vi "Process button press.vi"(0 "DataCluster in":T1={"JSONRead"={"ConfigurationFilePaths"={"Default JSON Path in"=path "", "Rack Controller Override JSON file path in"=path "", "Algorithm Overrride JSON file path in "=path ""}, "ConfigurationVariants"={"Default JSON \nVariant"=variant(cluster{"Inspection States":enum16{"PreSelect", "Back _Inspection", "Analytics", "Ready To Run", "Ready To Insert", "Enable All buttons", "Disable All Buttons", "Settings", "Select", "Stop", "Pause", "Inspect"}} {"Inspection States"=enum."PreSelect"}), "Algorithm Override\nJSON Variant"=variant(cluster{"Diagnostics States":enum16{"Enable All", "Camera Optics Fail", "Loading Bar", "Camera Optics", "Motor", "Arduino", "POST Done", "POST"}} {"Diagnostics States"=enum."Enable All"}), "Rack Controller Override\nJSON Variant"=variant(cluster{"Edit Limits":enum16{"Update List"}, "Enable Disable Measurements":enum16{"Back to Edit Tolerance"}, "Page Select":enum16{"Edit Tolerance Limits", "Enable Disable Buttons"}} {"Edit Limits"=enum."Update List", "Enable Disable Measurements"=enum."Back to Edit Tolerance", "Page Select"=enum."Edit Tolerance Limits"})}, "ConfigurationCluster"={"UIParameters"={"SpecificationVersion"="", "Title"="", "NumberOfImagesToBeDisplayed"=0.0, "ImageCountWindow"=0.0, "FontName"="", "FontSize"=0.0, "CustomerLogoFilePath"="", "ZentronLogoFilePath"="", "CompatibleSoftwareVersions"=[], "CameraLabelMapping"=[], "ImageIndicatorLayouts"=[], "SoftwareButtonLabels"={"SelectLabel"="", "RunLabel"="", "PauseLabel"="", "StopLabel"=""}, "DiagnosticsParameters"={"CameraOpticsDiagnostics"={"Label"="", "CameraLabelsList"=[]}, "ArduinoDiagnostics"={"Label"=""}, "MotorDiagnostics"={"Label"=""}, "ReelerMotor"={"Label"=""}, "TowerLampDiagnostics"={"Label"=""}, "TriggerSensor"={"Label"="", "SensorsList"=[]}, "HardwareButtonDiagnostics"={"Label"=""}, "MasterSampleDiagnostics"={"Label"=""}}, "DieIdParameters"={"DefaultDieId"="", "DieIdsList"=[]}, "EventReasonsList"={"Pause"=[], "Stop"=[], "FailPause"=[], "Ignored"=[], "DefaultEventReason"=""}, "StampingMachineIds"=[], "ErrorPopupStrings"=[]}}}, "Inspection"={"Inspection After Stop"=FALSE, "IsPaused"=FALSE, "Camera Names"=[], "Fail Array"=[], "Reel Number"=0, "Image details_init"=[], "LSL"=[], "USL"=[], "Max limits"={"Production max"=0, "Reel max"=0}, "parts List"=[], "#Racks"=0, "MeasurementNames"=[], "Reel complete"=FALSE, "Fail event reason list"=[]}, "Diagnostics"={"Selection Done?"=FALSE, "Diagnostics details"={"Diagnostics names"={"Main diagnostics"=[], "Sub diagnostics names"={"Camera optics"=[], "Trigger sensor"=[]}}, "Diagnostics labels"={"Main diagnostics"=[], "Sub diagnostics names"={"Camera optics"=[], "Trigger sensor"=[]}}}, "DiagnosticsFeatures"={"ArduinoDiagnostics"=FALSE, "MotorDiagnostics"=FALSE, "CameraOpticsDiagnostics"=FALSE, "ReelerMotor"=FALSE, "HardwareButtonDiagnostics"=FALSE, "TriggerSensor"=FALSE, "TowerLampDiagnostics"=FALSE, "MasterSampleDiagnostics"=FALSE}, "SelectedDiagnostics"=""}, "EditToleranceSettings"={"Input ListBox"={"Measurement Values"=[], "Cluster of Limits"={"LSL"=0.0, "USL"=0.0, "LCL"=0.0, "UCL"=0.0}, "Rack Selection"=enum."Both Racks", "M and N Array"=[], "Ticked Measurement Index"=[], "Measurements Enabled"=[], "Current Active Position"={"Horizontal"=0, "Vertical"=0}, "Current ticked measurement"=0.0}, "Saved?"=FALSE, "IsETLSelected"=FALSE, "IsPartSelected"=FALSE}, "ControlsIndicators"={"General"={"Main Tab"=refnum, "Inspection SubPanel_Inspection"=refnum, "Zen Logo_Inspection"=refnum, "SoftwareExit"=refnum, "Loading Bar VI Ref"=refnum, "Right Pane Tab"=refnum, "Image Reference array"=[], "Command tab"=refnum, "Inspection subTab control ref"=refnum, "SelectionCluster"={"ok"=refnum, "confirm"=refnum, "reset"=refnum, "change"=refnum, "TOTAL COUNT"=refnum, "REEL COUNT"=refnum, "PART NAME"=refnum, "VERIFIED"=refnum, "OPERATOR NAME"=refnum, "Select message"=refnum}, "Event  Reason  List"=refnum, "Event reason blink"=refnum, "Event reason switching tab"=refnum, "confirm_eventReason"=refnum}, "Inspection"={"Inspection Status"=refnum, "Run_Inspection"=refnum, "Pause_Inspection"=refnum, "Stop_Inspection"=refnum, "Settings_Inspection"=refnum, "Inspection Images VI Ref"=refnum, "Pass-Fail Indicator String"=refnum, "Analytics_Inspection"=refnum, "Label array"=[], "Analytics VI\nreference"=refnum, "Counts"=refnum, "Cards array"=refnum, "Counts array"=[]}, "Diagnostics"={"Diagnostics Tab"=refnum, "Dust indicator :"=refnum, "Logout_Diagnostics"=refnum, "CAMERA STATUS MESSAGE"=refnum, "BUZZER OFF"=refnum, "PAUSE"=refnum, "STOP"=refnum, "RUN"=refnum, "Current Diagnostics Status"=refnum, "Select a diagnostics"=refnum, "Diagnostics Status"=refnum, "Select a sub diagnostics"=refnum, "Optics img"=refnum, "Diagnostics Status\nString"=refnum}, "Edit Tolerance Limits"={"Tolerance Limits Listbox"=refnum, "Enable Disable"=refnum, "Cluster of limits"=refnum, "Thresholds limits"=refnum, "Update List"=refnum, "Save"=refnum, "Back_Edit Tolerance"=refnum, "logout"=refnum, "Select a part"=refnum, "Bias Correction"=refnum, "Linearity Correction"=refnum, "Select a Rack"=refnum, "ETS tab"=refnum, "Factory reset"=refnum, "Door\nPoka Yoke"=refnum, "Fail count reverse"=refnum, "ETL count error message"=refnum, "ETL help string"=refnum}, "Master sample"={"Master sample message"=refnum, "Master sample tab"=refnum, "Next"=refnum, "Repeat"=refnum, "Master sample part message"=refnum}}, "AdditionalFeatures"={"Cp Cpk details"={"CpCpkData"=[], "Cp Cpk popup"=refnum}, "Popup"={"Restore main tab"="", "Popup data"={"Loading bar data"={"Open?"=FALSE, "Display string"=""}, "Pop-up"={"Pop-up Type"=enum."Open Logo Display", "Title"="", "Message"="", "Button 1 Text"="", "Button 2 Text"="", "Show Close? T/F"=FALSE, "Title Blink? T/F"=FALSE, "Title Blink Colour"=0}}}, "DynamicImageHandling"={"Image update"=[], "RBCIA"=[], "ISIM"=[], "Camera labels list"=[], "Enable DIH?"=FALSE, "Init DIH params?"=FALSE}, "PageHandling"={"Previous State"={"Inspection"={"Inspection States"=enum."PreSelect"}, "Diagnostics"={"Diagnostics States"=enum."Enable All"}, "Edit Tolerance"={"Edit Limits"=enum."Update List", "Enable Disable Measurements"=enum."Back to Edit Tolerance", "Page Select"=enum."Edit Tolerance Limits"}, "Page Select"=enum."Edit Tolerance"}, "Current state"="", "Previous control access state"=""}, "Core"={"Current VI Reference"=refnum, "Close Panel on Exit?"=FALSE}, "SlaveLoopData"={"EnableShortKeyPress"=FALSE, "Point32"={"Horizontal"=0, "Vertical"=0}}, "Chosen event reason"="", "Master sample validation"={"Master sample general message"="", "Master sample part message"=""}, "Fail Ignore Count Reversal"={"Production ignored count"=0, "Reel ignored count"=0}}}, 1 "Label.Text":string, 5 "Send ClusterData":refnum<user-event>, 9 "Self Enqueuer":refnum<class "Message Enqueuer.lvclass">, 11 "error in (no error)":errorcluster, 12 "Caller Enqueuer":refnum<class "Message Enqueuer.lvclass">) -> (4 "DataCluster out":T1={"JSONRead"={"ConfigurationFilePaths"={"Default JSON Path in"=path "", "Rack Controller Override JSON file path in"=path "", "Algorithm Overrride JSON file path in "=path ""}, "ConfigurationVariants"={"Default JSON \nVariant"=variant(cluster{"Inspection States":enum16{"PreSelect", "Back _Inspection", "Analytics", "Ready To Run", "Ready To Insert", "Enable All buttons", "Disable All Buttons", "Settings", "Select", "Stop", "Pause", "Inspect"}} {"Inspection States"=enum."PreSelect"}), "Algorithm Override\nJSON Variant"=variant(cluster{"Diagnostics States":enum16{"Enable All", "Camera Optics Fail", "Loading Bar", "Camera Optics", "Motor", "Arduino", "POST Done", "POST"}} {"Diagnostics States"=enum."Enable All"}), "Rack Controller Override\nJSON Variant"=variant(cluster{"Edit Limits":enum16{"Update List"}, "Enable Disable Measurements":enum16{"Back to Edit Tolerance"}, "Page Select":enum16{"Edit Tolerance Limits", "Enable Disable Buttons"}} {"Edit Limits"=enum."Update List", "Enable Disable Measurements"=enum."Back to Edit Tolerance", "Page Select"=enum."Edit Tolerance Limits"})}, "ConfigurationCluster"={"UIParameters"={"SpecificationVersion"="", "Title"="", "NumberOfImagesToBeDisplayed"=0.0, "ImageCountWindow"=0.0, "FontName"="", "FontSize"=0.0, "CustomerLogoFilePath"="", "ZentronLogoFilePath"="", "CompatibleSoftwareVersions"=[], "CameraLabelMapping"=[], "ImageIndicatorLayouts"=[], "SoftwareButtonLabels"={"SelectLabel"="", "RunLabel"="", "PauseLabel"="", "StopLabel"=""}, "DiagnosticsParameters"={"CameraOpticsDiagnostics"={"Label"="", "CameraLabelsList"=[]}, "ArduinoDiagnostics"={"Label"=""}, "MotorDiagnostics"={"Label"=""}, "ReelerMotor"={"Label"=""}, "TowerLampDiagnostics"={"Label"=""}, "TriggerSensor"={"Label"="", "SensorsList"=[]}, "HardwareButtonDiagnostics"={"Label"=""}, "MasterSampleDiagnostics"={"Label"=""}}, "DieIdParameters"={"DefaultDieId"="", "DieIdsList"=[]}, "EventReasonsList"={"Pause"=[], "Stop"=[], "FailPause"=[], "Ignored"=[], "DefaultEventReason"=""}, "StampingMachineIds"=[], "ErrorPopupStrings"=[]}}}, "Inspection"={"Inspection After Stop"=FALSE, "IsPaused"=FALSE, "Camera Names"=[], "Fail Array"=[], "Reel Number"=0, "Image details_init"=[], "LSL"=[], "USL"=[], "Max limits"={"Production max"=0, "Reel max"=0}, "parts List"=[], "#Racks"=0, "MeasurementNames"=[], "Reel complete"=FALSE, "Fail event reason list"=[]}, "Diagnostics"={"Selection Done?"=FALSE, "Diagnostics details"={"Diagnostics names"={"Main diagnostics"=[], "Sub diagnostics names"={"Camera optics"=[], "Trigger sensor"=[]}}, "Diagnostics labels"={"Main diagnostics"=[], "Sub diagnostics names"={"Camera optics"=[], "Trigger sensor"=[]}}}, "DiagnosticsFeatures"={"ArduinoDiagnostics"=FALSE, "MotorDiagnostics"=FALSE, "CameraOpticsDiagnostics"=FALSE, "ReelerMotor"=FALSE, "HardwareButtonDiagnostics"=FALSE, "TriggerSensor"=FALSE, "TowerLampDiagnostics"=FALSE, "MasterSampleDiagnostics"=FALSE}, "SelectedDiagnostics"=""}, "EditToleranceSettings"={"Input ListBox"={"Measurement Values"=[], "Cluster of Limits"={"LSL"=0.0, "USL"=0.0, "LCL"=0.0, "UCL"=0.0}, "Rack Selection"=enum."Both Racks", "M and N Array"=[], "Ticked Measurement Index"=[], "Measurements Enabled"=[], "Current Active Position"={"Horizontal"=0, "Vertical"=0}, "Current ticked measurement"=0.0}, "Saved?"=FALSE, "IsETLSelected"=FALSE, "IsPartSelected"=FALSE}, "ControlsIndicators"={"General"={"Main Tab"=refnum, "Inspection SubPanel_Inspection"=refnum, "Zen Logo_Inspection"=refnum, "SoftwareExit"=refnum, "Loading Bar VI Ref"=refnum, "Right Pane Tab"=refnum, "Image Reference array"=[], "Command tab"=refnum, "Inspection subTab control ref"=refnum, "SelectionCluster"={"ok"=refnum, "confirm"=refnum, "reset"=refnum, "change"=refnum, "TOTAL COUNT"=refnum, "REEL COUNT"=refnum, "PART NAME"=refnum, "VERIFIED"=refnum, "OPERATOR NAME"=refnum, "Select message"=refnum}, "Event  Reason  List"=refnum, "Event reason blink"=refnum, "Event reason switching tab"=refnum, "confirm_eventReason"=refnum}, "Inspection"={"Inspection Status"=refnum, "Run_Inspection"=refnum, "Pause_Inspection"=refnum, "Stop_Inspection"=refnum, "Settings_Inspection"=refnum, "Inspection Images VI Ref"=refnum, "Pass-Fail Indicator String"=refnum, "Analytics_Inspection"=refnum, "Label array"=[], "Analytics VI\nreference"=refnum, "Counts"=refnum, "Cards array"=refnum, "Counts array"=[]}, "Diagnostics"={"Diagnostics Tab"=refnum, "Dust indicator :"=refnum, "Logout_Diagnostics"=refnum, "CAMERA STATUS MESSAGE"=refnum, "BUZZER OFF"=refnum, "PAUSE"=refnum, "STOP"=refnum, "RUN"=refnum, "Current Diagnostics Status"=refnum, "Select a diagnostics"=refnum, "Diagnostics Status"=refnum, "Select a sub diagnostics"=refnum, "Optics img"=refnum, "Diagnostics Status\nString"=refnum}, "Edit Tolerance Limits"={"Tolerance Limits Listbox"=refnum, "Enable Disable"=refnum, "Cluster of limits"=refnum, "Thresholds limits"=refnum, "Update List"=refnum, "Save"=refnum, "Back_Edit Tolerance"=refnum, "logout"=refnum, "Select a part"=refnum, "Bias Correction"=refnum, "Linearity Correction"=refnum, "Select a Rack"=refnum, "ETS tab"=refnum, "Factory reset"=refnum, "Door\nPoka Yoke"=refnum, "Fail count reverse"=refnum, "ETL count error message"=refnum, "ETL help string"=refnum}, "Master sample"={"Master sample message"=refnum, "Master sample tab"=refnum, "Next"=refnum, "Repeat"=refnum, "Master sample part message"=refnum}}, "AdditionalFeatures"={"Cp Cpk details"={"CpCpkData"=[], "Cp Cpk popup"=refnum}, "Popup"={"Restore main tab"="", "Popup data"={"Loading bar data"={"Open?"=FALSE, "Display string"=""}, "Pop-up"={"Pop-up Type"=enum."Open Logo Display", "Title"="", "Message"="", "Button 1 Text"="", "Button 2 Text"="", "Show Close? T/F"=FALSE, "Title Blink? T/F"=FALSE, "Title Blink Colour"=0}}}, "DynamicImageHandling"={"Image update"=[], "RBCIA"=[], "ISIM"=[], "Camera labels list"=[], "Enable DIH?"=FALSE, "Init DIH params?"=FALSE}, "PageHandling"={"Previous State"={"Inspection"={"Inspection States"=enum."PreSelect"}, "Diagnostics"={"Diagnostics States"=enum."Enable All"}, "Edit Tolerance"={"Edit Limits"=enum."Update List", "Enable Disable Measurements"=enum."Back to Edit Tolerance", "Page Select"=enum."Edit Tolerance Limits"}, "Page Select"=enum."Edit Tolerance"}, "Current state"="", "Previous control access state"=""}, "Core"={"Current VI Reference"=refnum, "Close Panel on Exit?"=FALSE}, "SlaveLoopData"={"EnableShortKeyPress"=FALSE, "Point32"={"Horizontal"=0, "Vertical"=0}}, "Chosen event reason"="", "Master sample validation"={"Master sample general message"="", "Master sample part message"=""}, "Fail Ignore Count Reversal"={"Production ignored count"=0, "Reel ignored count"=0}}}, 15 "error out":errorcluster)   [LabVIEW 2019, in "ZenGage v3.0 UI.lvclass"]
uses:
  ZenGage v3.0 UI.lvclass
  <vilib>/ActorFramework/Message Enqueuer/Message Priority.ctl
  <vilib>/ActorFramework/Message Enqueuer/Message Enqueuer.lvclass
  User Interface Messages/User Interface messages/Call function_UI Msg/ButtonPress_UI.lvclass
  Common/Controls/Acknowledgement.ctl
  Type Definitions/General/OutputDetails.ctl
  Type Definitions/General/Output choice.ctl
  Type Definitions/General/UI States(UI button enable disable).ctl
  Type Definitions/Controls and Indicators/Select a part (combobox).ctl
  Type Definitions/Controls and Indicators/EDL control references.ctl
  Type Definitions/Controls and Indicators/Diagnostics control referencs.ctl
  Type Definitions/Controls and Indicators/Inspection control references.ctl
  Type Definitions/Controls and Indicators/General_Control references.ctl
  Type Definitions/Controls and Indicators/Controls and Indicators Cluster.ctl
  Type Definitions/JSON Read/UI JSON read cluster.ctl
  Type Definitions/General/JSONRead.ctl
  Type Definitions/Inspection/Inspection Cluster.ctl
  Type Definitions/Diagnostics/Diagnostics(Cluster).ctl
  Type Definitions/Edit tolerance settings/Rack Selection.ctl
  <vilib>/Utility/miscctls.llb/LVPoint32TypeDef.ctl
  Type Definitions/Edit tolerance settings/Edit Tolerance Input.ctl
  Type Definitions/Edit tolerance settings/Edit Tolerance Overall Cluster.ctl
  Common/Controls/Pop-up Input.ctl
  Type Definitions/General/UIDataCluster.ctl
  Type Definitions/General/Master sample references.ctl
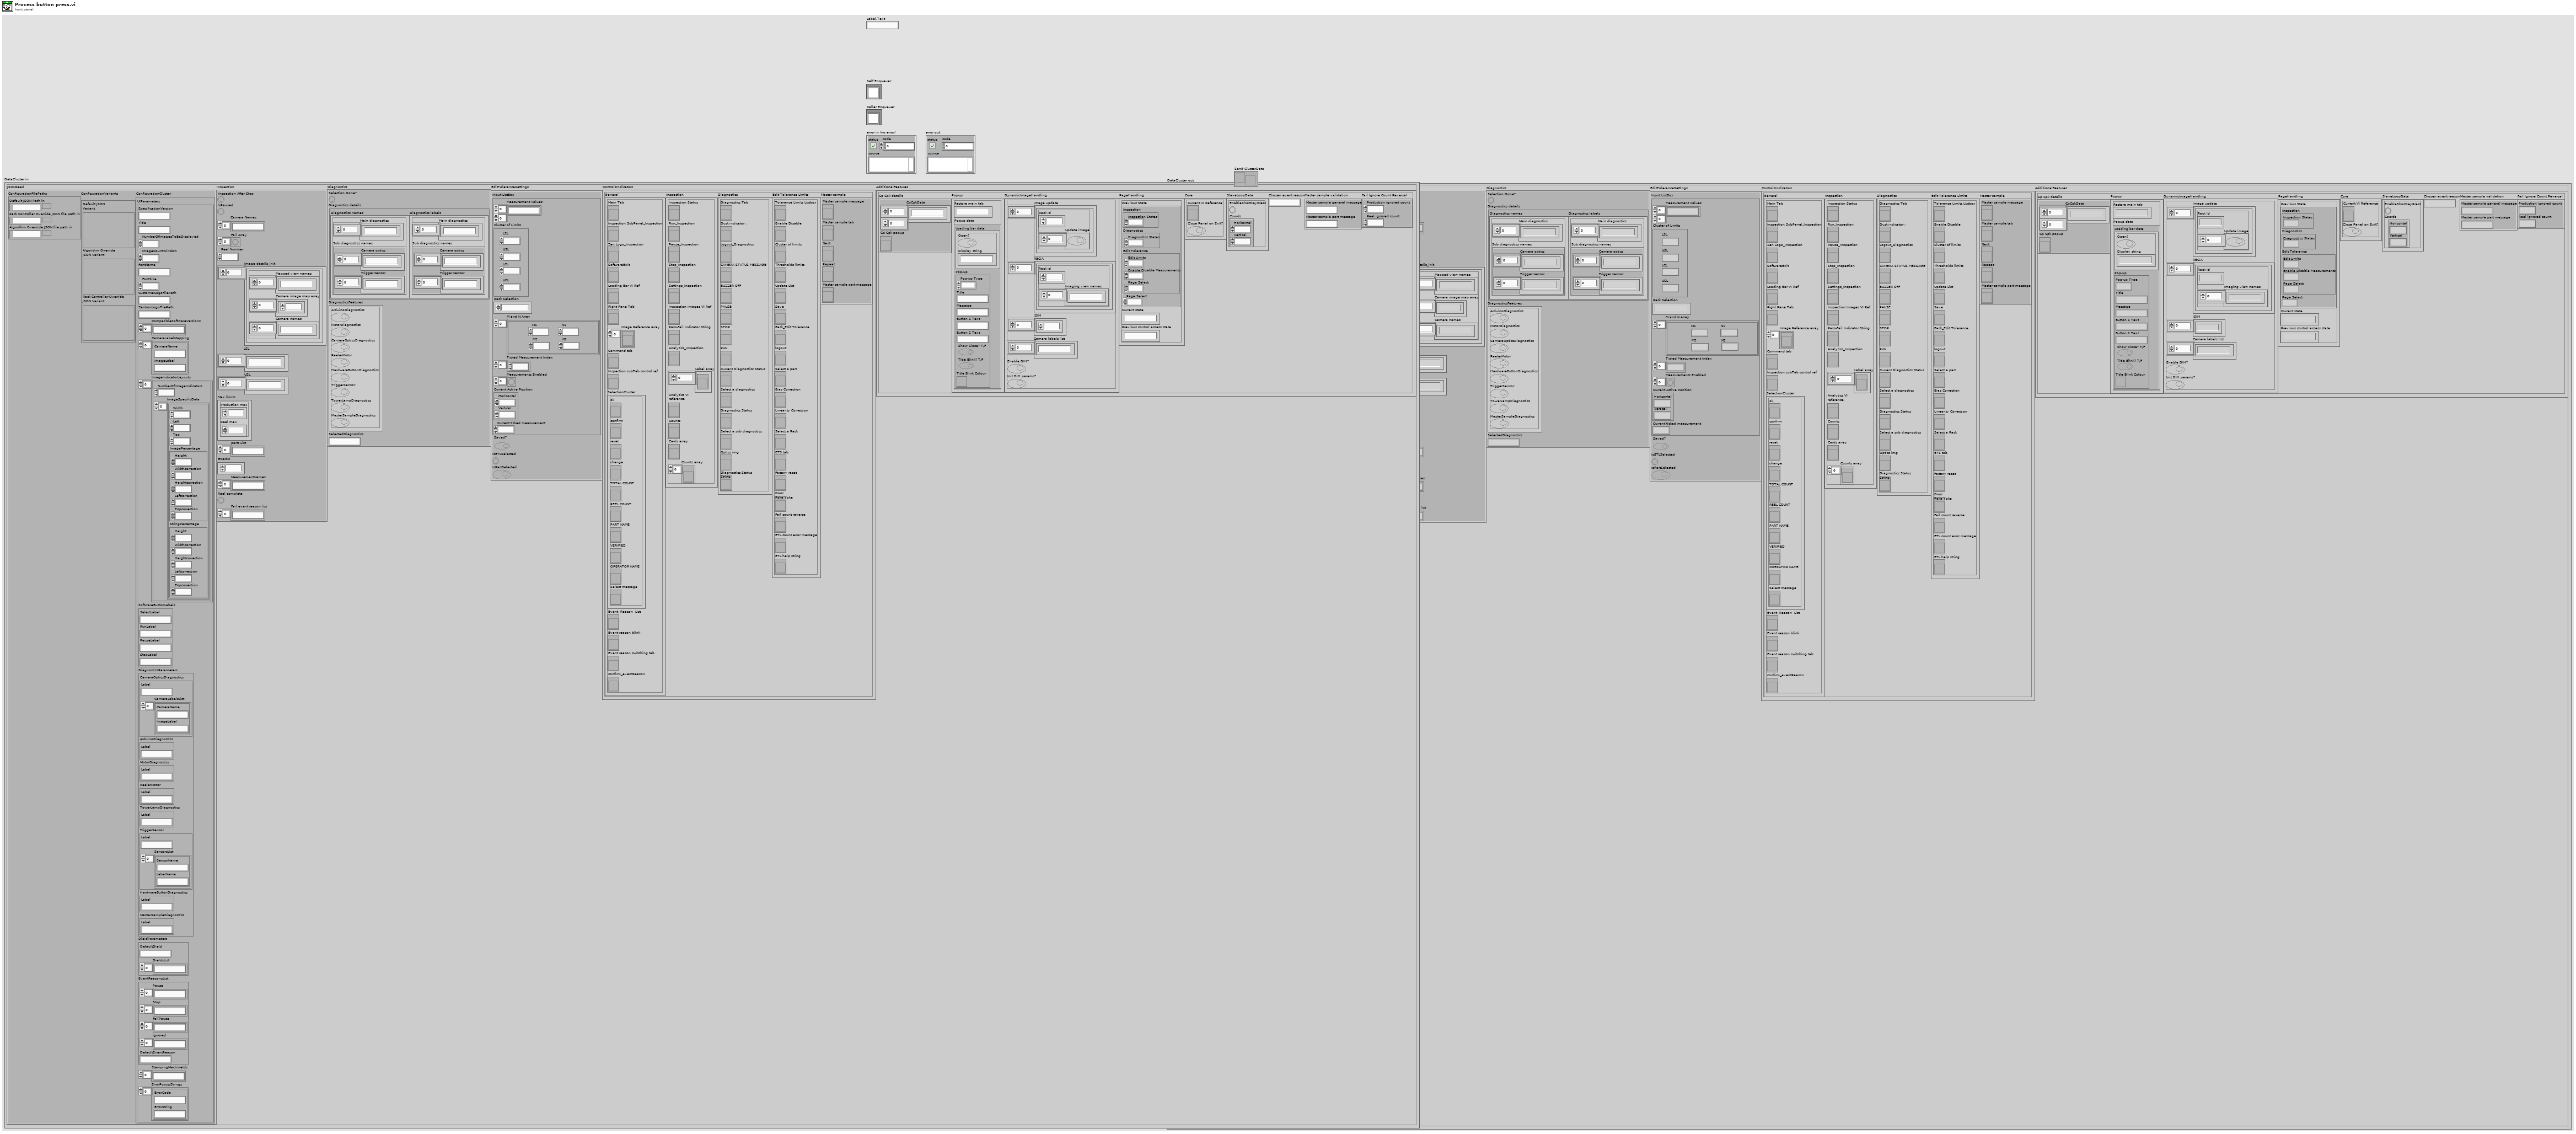
[diagram p1: front panel]
types:
  T1 = typedef "UIDataCluster.ctl" = cluster{"JSONRead":T2, "Inspection":T4, "Diagnostics":T5, "EditToleranceSettings":T6, "ControlsIndicators":T10, "AdditionalFeatures":cluster{"Cp Cpk details":cluster{"CpCpkData":string[][], "Cp Cpk popup":refnum<vi>}, "Popup":cluster{"Restore main tab":string, "Popup data":cluster{"Loading bar data":cluster{"Open?":bool, "Display string":string}, "Pop-up":T16}}, "DynamicImageHandling":cluster{"Image update":cluster{"Rack Id":i32, "Update image":bool[]}[], "RBCIA":cluster{"Rack Id":u8, "Imaging view names":string[]}[], "ISIM":u8[], "Camera labels list":string[], "Enable DIH?":bool, "Init DIH params?":bool}, "PageHandling":cluster{"Previous State":T17, "Current state":string, "Previous control access state":string}, "Core":cluster{"Current VI Reference":refnum<vi>, "Close Panel on Exit?":bool}, "SlaveLoopData":cluster{"EnableShortKeyPress":bool, "Point32":T9}, "Chosen event reason":string, "Master sample validation":cluster{"Master sample general message":string, "Master sample part message":string}, "Fail Ignore Count Reversal":cluster{"Production ignored count":u64, "Reel ignored count":u64}}}
  T2 = typedef "ZenGage v3.0 UI.lvclass/JSONRead.ctl" = cluster{"ConfigurationFilePaths":cluster{"Default JSON Path in":path, "Rack Controller Override JSON file path in":path, "Algorithm Overrride JSON file path in ":path}, "ConfigurationVariants":cluster{"Default JSON \nVariant":variant, "Algorithm Override\nJSON Variant":variant, "Rack Controller Override\nJSON Variant":variant}, "ConfigurationCluster":T3}
  T3 = typedef "ZenGage v3.0 UI.lvclass/UI JSON read cluster.ctl" = cluster{"UIParameters":cluster{"SpecificationVersion":string, "Title":string, "NumberOfImagesToBeDisplayed":dbl, "ImageCountWindow":dbl, "FontName":string, "FontSize":dbl, "CustomerLogoFilePath":string, "ZentronLogoFilePath":string, "CompatibleSoftwareVersions":string[], "CameraLabelMapping":cluster{"CameraName":string, "ImageLabel":string}[], "ImageIndicatorLayouts":cluster{"NumberOfImageIndicators":dbl, "ImageSpecificData":cluster{"Width":dbl, "Left":dbl, "Top":dbl, "ImagePercentage":cluster{"Height":dbl, "Widthcorrection":i64, "Heightcorrection":i64, "Leftcorrection":dbl, "Topcorrection":dbl}, "StringPercentage":cluster{"Height":dbl, "Widthcorrection":i64, "Heightcorrection":dbl, "Leftcorrection":dbl, "Topcorrection":dbl}}[]}[], "SoftwareButtonLabels":cluster{"SelectLabel":string, "RunLabel":string, "PauseLabel":string, "StopLabel":string}, "DiagnosticsParameters":cluster{"CameraOpticsDiagnostics":cluster{"Label":string, "CameraLabelsList":cluster{"CameraName":string, "ImageLabel":string}[]}, "ArduinoDiagnostics":cluster{"Label":string}, "MotorDiagnostics":cluster{"Label":string}, "ReelerMotor":cluster{"Label":string}, "TowerLampDiagnostics":cluster{"Label":string}, "TriggerSensor":cluster{"Label":string, "SensorsList":cluster{"SensorName":string, "LabelName":string}[]}, "HardwareButtonDiagnostics":cluster{"Label":string}, "MasterSampleDiagnostics":cluster{"Label":string}}, "DieIdParameters":cluster{"DefaultDieId":string, "DieIdsList":string[]}, "EventReasonsList":cluster{"Pause":string[], "Stop":string[], "FailPause":string[], "Ignored":string[], "DefaultEventReason":string}, "StampingMachineIds":string[], "ErrorPopupStrings":cluster{"ErrorCode":string, "ErrorString":string}[]}}
  T4 = typedef "ZenGage v3.0 UI.lvclass/Inspection Cluster.ctl" = cluster{"Inspection After Stop":bool, "IsPaused":bool, "Camera Names":string[], "Fail Array":bool[], "Reel Number":u32, "Image details_init":cluster{"Mapped view names":string[], "Camera image map array":i32[], "Camera names":string[]}[], "LSL":string[], "USL":string[], "Max limits":cluster{"Production max":u64, "Reel max":u64}, "parts List":string[], "#Racks":u8, "MeasurementNames":string[], "Reel complete":bool, "Fail event reason list":string[]}
  T5 = typedef "ZenGage v3.0 UI.lvclass/Diagnostics(Cluster).ctl" = cluster{"Selection Done?":bool, "Diagnostics details":cluster{"Diagnostics names":cluster{"Main diagnostics":string[], "Sub diagnostics names":cluster{"Camera optics":string[], "Trigger sensor":string[]}}, "Diagnostics labels":cluster{"Main diagnostics":string[], "Sub diagnostics names":cluster{"Camera optics":string[], "Trigger sensor":string[]}}}, "DiagnosticsFeatures":cluster{"ArduinoDiagnostics":bool, "MotorDiagnostics":bool, "CameraOpticsDiagnostics":bool, "ReelerMotor":bool, "HardwareButtonDiagnostics":bool, "TriggerSensor":bool, "TowerLampDiagnostics":bool, "MasterSampleDiagnostics":bool}, "SelectedDiagnostics":string}
  T6 = typedef "ZenGage v3.0 UI.lvclass/Edit Tolerance Overall Cluster.ctl" = cluster{"Input ListBox":T7, "Saved?":bool, "IsETLSelected":bool, "IsPartSelected":bool}
  T7 = typedef "ZenGage v3.0 UI.lvclass/Edit Tolerance Input.ctl" = cluster{"Measurement Values":string[][], "Cluster of Limits":cluster{"LSL":dbl, "USL":dbl, "LCL":dbl, "UCL":dbl}, "Rack Selection":T8, "M and N Array":cluster{"M1":u64, "M2":u64, "N1":u64, "N2":u64}[], "Ticked Measurement Index":u32[], "Measurements Enabled":bool[], "Current Active Position":T9, "Current ticked measurement":dbl}
  T8 = typedef "ZenGage v3.0 UI.lvclass/Rack Selection.ctl" = enum16{"Both Racks", "Rack 2", "Rack 1"}
  T9 = typedef "LVPoint32TypeDef.ctl" = cluster{"Horizontal":i32, "Vertical":i32}
  T10 = typedef "ZenGage v3.0 UI.lvclass/Controls and Indicators Cluster.ctl" = cluster{"General":T11, "Inspection":T12, "Diagnostics":T13, "Edit Tolerance Limits":T14, "Master sample":T15}
  T11 = typedef "ZenGage v3.0 UI.lvclass/General_Control references.ctl" = cluster{"Main Tab":refnum<vi>, "Inspection SubPanel_Inspection":refnum<vi>, "Zen Logo_Inspection":refnum<vi>, "SoftwareExit":refnum<vi>, "Loading Bar VI Ref":refnum<vi>, "Right Pane Tab":refnum<vi>, "Image Reference array":refnum<vi>[], "Command tab":refnum<vi>, "Inspection subTab control ref":refnum<vi>, "SelectionCluster":cluster{"ok":refnum<vi>, "confirm":refnum<vi>, "reset":refnum<vi>, "change":refnum<vi>, "TOTAL COUNT":refnum<vi>, "REEL COUNT":refnum<vi>, "PART NAME":refnum<vi>, "VERIFIED":refnum<vi>, "OPERATOR NAME":refnum<vi>, "Select message":refnum<vi>}, "Event  Reason  List":refnum<vi>, "Event reason blink":refnum<vi>, "Event reason switching tab":refnum<vi>, "confirm_eventReason":refnum<vi>}
  T12 = typedef "ZenGage v3.0 UI.lvclass/Inspection control references.ctl" = cluster{"Inspection Status":refnum<vi>, "Run_Inspection":refnum<vi>, "Pause_Inspection":refnum<vi>, "Stop_Inspection":refnum<vi>, "Settings_Inspection":refnum<vi>, "Inspection Images VI Ref":refnum<vi>, "Pass-Fail Indicator String":refnum<vi>, "Analytics_Inspection":refnum<vi>, "Label array":refnum<vi>[], "Analytics VI\nreference":refnum<vi>, "Counts":refnum<vi>, "Cards array":refnum<vi>, "Counts array":refnum<vi>[]}
  T13 = typedef "ZenGage v3.0 UI.lvclass/Diagnostics control referencs.ctl" = cluster{"Diagnostics Tab":refnum<vi>, "Dust indicator :":refnum<vi>, "Logout_Diagnostics":refnum<vi>, "CAMERA STATUS MESSAGE":refnum<vi>, "BUZZER OFF":refnum<vi>, "PAUSE":refnum<vi>, "STOP":refnum<vi>, "RUN":refnum<vi>, "Current Diagnostics Status":refnum<vi>, "Select a diagnostics":refnum<vi>, "Diagnostics Status":refnum<vi>, "Select a sub diagnostics":refnum<vi>, "Optics img":refnum<vi>, "Diagnostics Status\nString":refnum<vi>}
  T14 = typedef "ZenGage v3.0 UI.lvclass/EDL control references.ctl" = cluster{"Tolerance Limits Listbox":refnum<vi>, "Enable Disable":refnum<vi>, "Cluster of limits":refnum<vi>, "Thresholds limits":refnum<vi>, "Update List":refnum<vi>, "Save":refnum<vi>, "Back_Edit Tolerance":refnum<vi>, "logout":refnum<vi>, "Select a part":refnum<vi>, "Bias Correction":refnum<vi>, "Linearity Correction":refnum<vi>, "Select a Rack":refnum<vi>, "ETS tab":refnum<vi>, "Factory reset":refnum<vi>, "Door\nPoka Yoke":refnum<vi>, "Fail count reverse":refnum<vi>, "ETL count error message":refnum<vi>, "ETL help string":refnum<vi>}
  T15 = typedef "Master sample references.ctl" = cluster{"Master sample message":refnum<vi>, "Master sample tab":refnum<vi>, "Next":refnum<vi>, "Repeat":refnum<vi>, "Master sample part message":refnum<vi>}
  T16 = typedef "Pop-up Input.ctl" = cluster{"Pop-up Type":enum16{"Open Logo Display", "Close Logo Display", "Open Loading Bar", "Close Loading Bar", "Open Alert Display", "Close Alert Display", "One button dialog box", "Two button dialog box", "User Authentication"}, "Title":string, "Message":string, "Button 1 Text":string, "Button 2 Text":string, "Show Close? T/F":bool, "Title Blink? T/F":bool, "Title Blink Colour":u32}
  T17 = typedef "ZenGage v3.0 UI.lvclass/UI States(UI button enable disable).ctl" = cluster{"Inspection":cluster{"Inspection States":enum16{"PreSelect", "Back _Inspection", "Analytics", "Ready To Run", "Ready To Insert", "Enable All buttons", "Disable All Buttons", "Settings", "Select", "Stop", "Pause", "Inspect"}}, "Diagnostics":cluster{"Diagnostics States":enum16{"Enable All", "Camera Optics Fail", "Loading Bar", "Camera Optics", "Motor", "Arduino", "POST Done", "POST"}}, "Edit Tolerance":cluster{"Edit Limits":enum16{"Update List"}, "Enable Disable Measurements":enum16{"Back to Edit Tolerance"}, "Page Select":enum16{"Edit Tolerance Limits", "Enable Disable Buttons"}}, "Page Select":enum16{"Edit Tolerance", "Diagnostics", "Inspection"}}
  T18 = typedef "ZenGage v3.0 UI.lvclass/Output choice.ctl" = enum16{"SendIgnoredFailCount", "SendPartDetails", "ButtonPress", "SendAcknowledgement", "InitiateCameraDiagnostics", "InitiateSensorDiagnostics", "SendPopupResponse", "SendEventReasonResponse", "SendErrorDetails"}
  T19 = typedef "ZenGage v3.0 UI.lvclass/OutputDetails.ctl" = cluster{"Acknowledgement_SM":T20, "Button name":string, "PartDetails":cluster{"PartName":string, "ConnectorsInReel":u64, "TotalCounts":u64, "OperatorName":string, "StampingMachineID":u32}, "SensorName":string, "CameraName":string, "PopupFeedbackDetails":cluster{"Pop-up Type":enum16{"Open Logo Display", "Close Logo Display", "Open Loading Bar", "Close Loading Bar", "Open Alert Display", "Close Alert Display", "One button dialog box", "Two button dialog box", "User Authentication"}, "Message":string, "Pressed Button":string}, "EventResponse":string, "ErrorMessage":string, "FailCountIgnore":cluster{"ReelIgnoreCount":u64, "ProductionIgnoreCount":u64}}
  T20 = typedef "Acknowledgement.ctl" = cluster{"Enqueuer":refnum<class "Message Enqueuer.lvclass">, "VIReference":refnum<vi>, "VIName":string}
  T21 = enum8{"Enabled", "Disabled", "Disabled and Grayed Out"}
  T22 = typedef "Actor Framework.lvlib/Message Enqueuer.lvclass/Message Priority.ctl" = enum16{"Low", "Normal", "High"}
  T23 = enum32{"Edit Tolerance Limits1", "Inspection", "Master sample", "Diagnostics"}
  T24 = enum32{"Arduino Motor", "Sensor trigger", "Hardware Button", "Camera Optics"}
  T25 = cluster{"IsSelected":bool, "IsSaved":bool, "Previous State":T17, "IsPaused":bool, "IsETSelected":bool, "Measurements Enabled":bool[]}
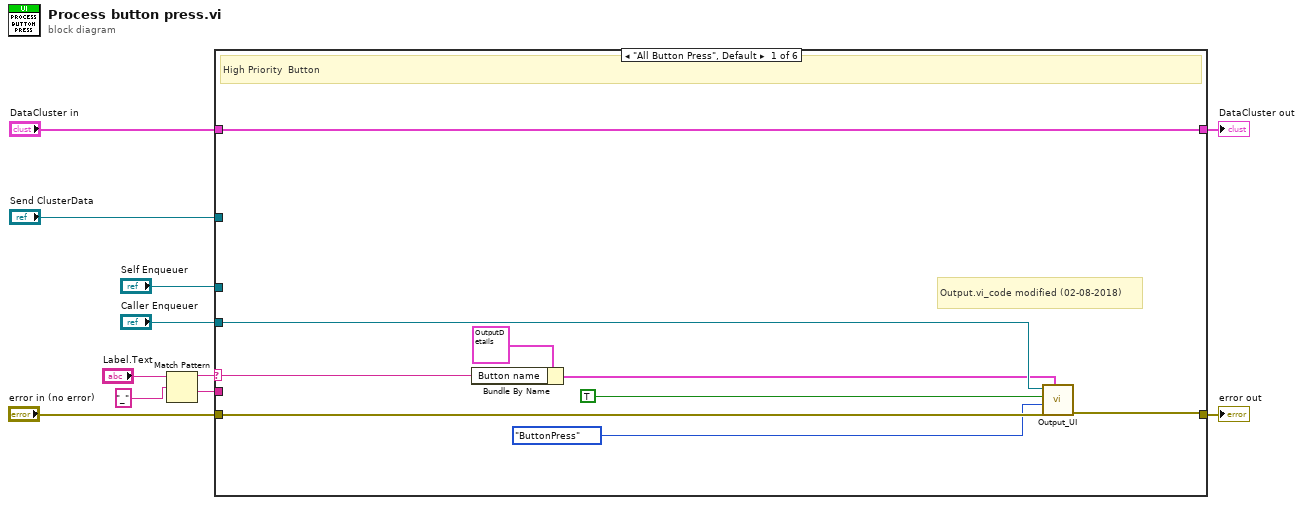
[diagram p0: block diagram]
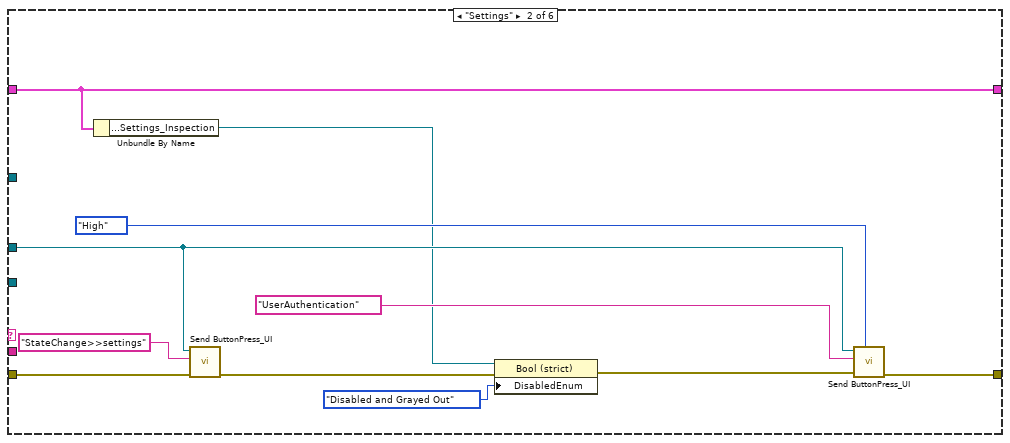
[diagram p2: hidden frame]
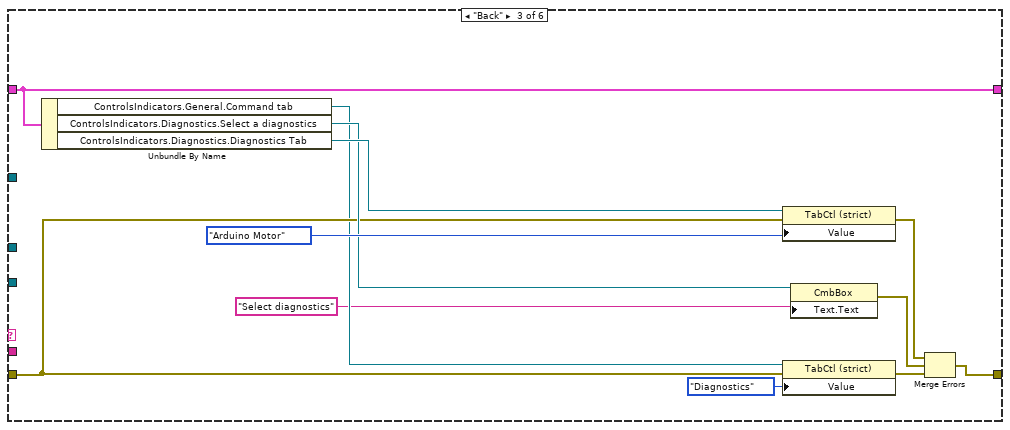
[diagram p3: hidden frame]
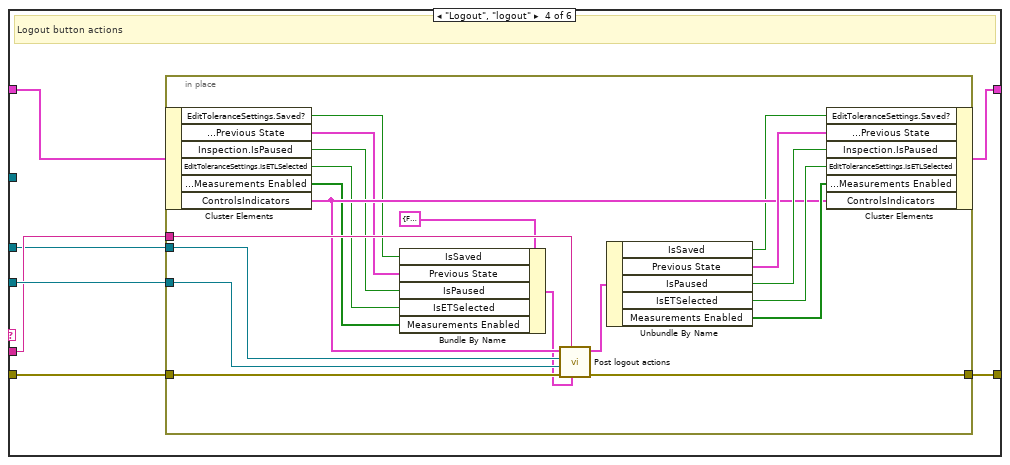
[diagram p4: hidden frame]
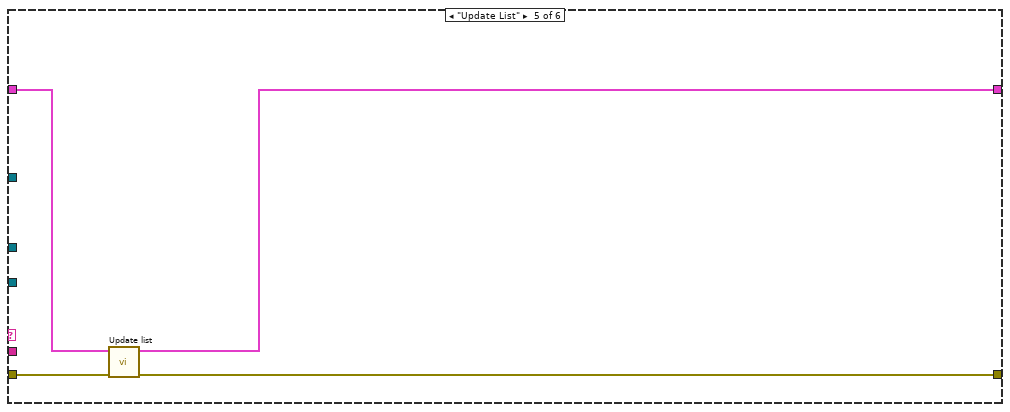
[diagram p5: hidden frame]
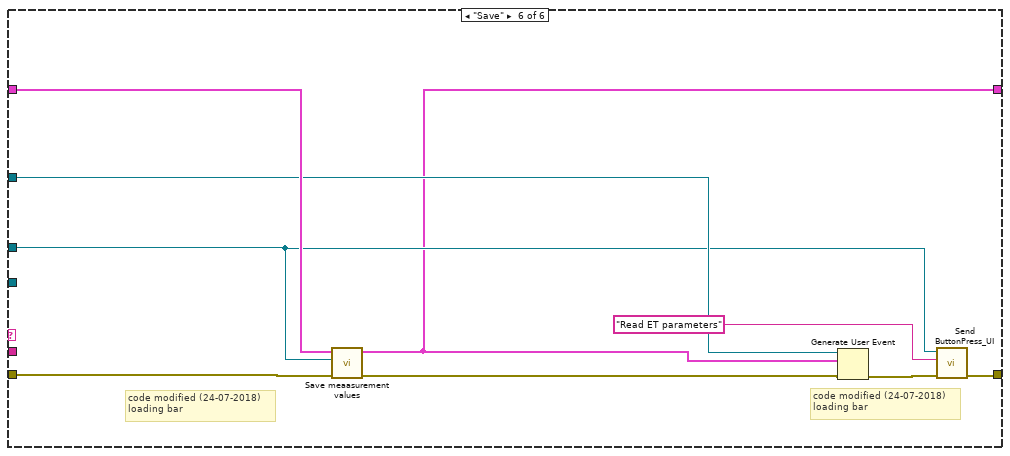
[diagram p6: hidden frame]
diagram:
  n1 = Match Pattern(string="Label.Text", regular expression="_") -> (before substring=w7:string, after substring=w9:string)  [unwired: 1 in, 2 out]
  n2 = case shown="\"All Button Press\", Default" w7 {
    selector: w7 -> [w16 _ _ _ _ _]
    tunnel: "Caller Enqueuer" -> [w18 _ _ w50 _ _]
    tunnel: "error in (no error)" -> [w20 w29 w40 w47 w71 w82]
    tunnel: [w19 w31 w38 w49 w72 w77] -> w6
    tunnel: "DataCluster in" -> [w12 w25 w33 w45 w73 w80]
    tunnel: w9 -> [_ _ _ w48 _ _]
    tunnel: "Self Enqueuer" -> [_ w28 _ w46 _ w76]
    tunnel: [w12 w25 w33 w44 w70 w74] -> w2
    tunnel: "Send ClusterData" -> [_ _ _ _ _ w79]
    frame "All Button Press", Default {
      # "Output.vi_code modified (02-08-2018)"
      # "High Priority  Button"
      n3 = Bundle By Name(cluster=T19 {"Acknowledgement_SM"={"Enqueuer"=refnum, "VIReference"=refnum, "VIName"=""}, "Button name"="", "PartDetails"={"PartName"="", "ConnectorsInReel"=0, "TotalCounts"=0, "OperatorName"="", "StampingMachineID"=0}, "SensorName"="", "CameraName"="", "PopupFeedbackDetails"={"Pop-up Type"=enum."Open Logo Display", "Message"="", "Pressed Button"=""}, "EventResponse"="", "ErrorMessage"="", "FailCountIgnore"={"ReelIgnoreCount"=0, "ProductionIgnoreCount"=0}} ("OutputDetails"), "Button name"=w16) -> (w15:T19)
      n4 = call "Output_UI.vi"("OutputDetails"=w15, "error in"=w20, "Functionality"=Output_choice."ButtonPress", "Testbench"=TRUE, "SMEnqueuer"=w18) -> ("error out"=w19:errorcluster)  [unwired: 6 in]
    }
    frame "Settings" {
      n5 = Unbundle By Name(w25) -> ("ControlsIndicators.Inspection.Settings_Inspection"=w22:refnum<vi>)
      n6 = call "Send ButtonPress_UI.vi"("error in (no error)"=w29, "FunctionalityName"="StateChange>>settings", "Message Enqueuer"=w28) -> ("error out"=w24:errorcluster)  [unwired: 7 in, 1 out]
      n7 = property class="Bool (strict)"(reference=w22, error in=w24, "DisabledEnum"=T21."Disabled and Grayed Out" ("Disabled")) -> (error out=w23:errorcluster)  [unwired: 1 out]
      n8 = call "Send ButtonPress_UI.vi"("Message Priority (Normal)"=Message_Priority."High", "error in (no error)"=w23, "FunctionalityName"="UserAuthentication" ("Functionality name"), "Message Enqueuer"=w28) -> ("error out"=w31:errorcluster)  [unwired: 6 in, 1 out]
    }
    frame "Back" {
      n9 = Unbundle By Name(w33) -> ("ControlsIndicators.General.Command tab"=w39:refnum<vi>, "ControlsIndicators.Diagnostics.Select a diagnostics"=w41:refnum<vi>, "ControlsIndicators.Diagnostics.Diagnostics Tab"=w43:refnum<vi>)
      n10 = property class="TabCtl (strict)"(reference=w43, error in=w40, "Value"=T24."Arduino Motor") -> (error out=w36:errorcluster)  [unwired: 1 out]
      n11 = property class="TabCtl (strict)"(reference=w39, error in=w40, "Value"=T23."Diagnostics") -> (error out=w34:errorcluster)  [unwired: 1 out]
      n12 = property class="CmbBox"(reference=w41, "Text.Text"="Select diagnostics") -> (error out=w35:errorcluster)  [unwired: 1 in, 1 out]
      n13 = Merge Errors(w36, w35, w34) -> (w38:errorcluster)
    }
    frame "Logout", "logout" {
      # "Logout button actions"
      n14 = in-place {
        in-place-border: w50 -> [w69]
        in-place-border: [w68] -> w49
        in-place-border: w48 -> [w67]
        in-place-border: w47 -> [w66]
        in-place-border: w46 -> [w65]
        n15 = in-place-cluster #1(w45) -> ("EditToleranceSettings.Saved?"=w57:bool, "AdditionalFeatures.PageHandling.Previous State"=w56:T17, "Inspection.IsPaused"=w55:bool, "EditToleranceSettings.IsETLSelected"=w54:bool, "EditToleranceSettings.Input ListBox.Measurements Enabled"=w53:bool[], "ControlsIndicators"=w59:T10)
        n16 = Bundle By Name(cluster=T25 {"IsSelected"=FALSE, "IsSaved"=FALSE, "Previous State"={"Inspection"={"Inspection States"=enum."PreSelect"}, "Diagnostics"={"Diagnostics States"=enum."Enable All"}, "Edit Tolerance"={"Edit Limits"=enum."Update List", "Enable Disable Measurements"=enum."Back to Edit Tolerance", "Page Select"=enum."Edit Tolerance Limits"}, "Page Select"=enum."Edit Tolerance"}, "IsPaused"=FALSE, "IsETSelected"=FALSE, "Measurements Enabled"=[]} ("Cluster out"), "IsSaved"=w57, "Previous State"=w56, "IsPaused"=w55, "IsETSelected"=w54, "Measurements Enabled"=w53) -> (w52:T25)
        n17 = call "Post logout actions.vi"("Cluster out"=w52, "Label.Text"=w67, "error in (no error)"=w66, "Caller Enqueuer"=w69, "Self Enqueuer"=w65, "ControlsIndicators"=w59) -> ("error out"=w68:errorcluster, "Cluster out"=w64:T25)  [unwired: 4 in]
        n18 = Unbundle By Name(w64) -> ("IsSaved"=w51:bool, "Previous State"=w63:T17, "IsPaused"=w62:bool, "IsETSelected"=w61:bool, "Measurements Enabled"=w60:bool[])
        n19 = in-place-cluster #1("EditToleranceSettings.Saved?"=w51, "AdditionalFeatures.PageHandling.Previous State"=w63, "Inspection.IsPaused"=w62, "EditToleranceSettings.IsETLSelected"=w61, "EditToleranceSettings.Input ListBox.Measurements Enabled"=w60, "ControlsIndicators"=w59) -> (w44:T1)
      }
    }
    frame "Update List" {
      n20 = call "Update list.vi"("error in (no error)"=w71, "ZenGage v3.0 UI in"=w73) -> ("error out"=w72:errorcluster, "ZenGage v3.0 UI out"=w70:T1)  [unwired: 8 in]
    }
    frame "Save" {
      # "code modified (24-07-2018)\nloading bar"
      # "code modified (24-07-2018)\nloading bar"
      n21 = call "Save meaasurement values.vi"("error in (no error)"=w82, "User interface enqueuer"=w76, "DataCluster in"=w80) -> ("error out"=w81:errorcluster, "DatCluster out"=w74:T1)  [unwired: 7 in]
      n22 = Generate User Event(user event=w79, event data cluster=w74, error in=w81) -> (error out=w78:errorcluster)  [unwired: 1 in, 1 out]
      n23 = call "Send ButtonPress_UI.vi"("error in (no error)"=w78, "FunctionalityName"="Read ET parameters", "Message Enqueuer"=w76) -> ("error out"=w77:errorcluster)  [unwired: 7 in, 1 out]
    }
  }
  "DataCluster out" <- w2
  "error out" <- w6
